vi "Extract Parameters from Comments.vi"(10 "Scan names":string[](array[string]), 11 "Comments":string) -> (1 "Numeric 3":dbl, 2 "Numeric 2":dbl, 3 "Numeric 1":dbl)   [LabVIEW 2020, in "Retrieve and Visualize.lvclass"]
uses:
  Retrieve and Visualize.lvclass
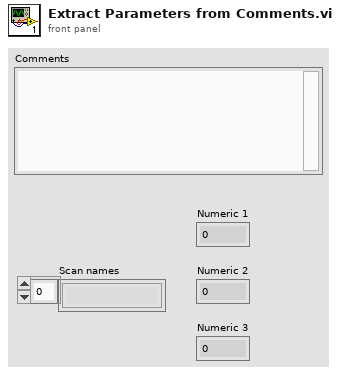
[diagram p1: front panel]
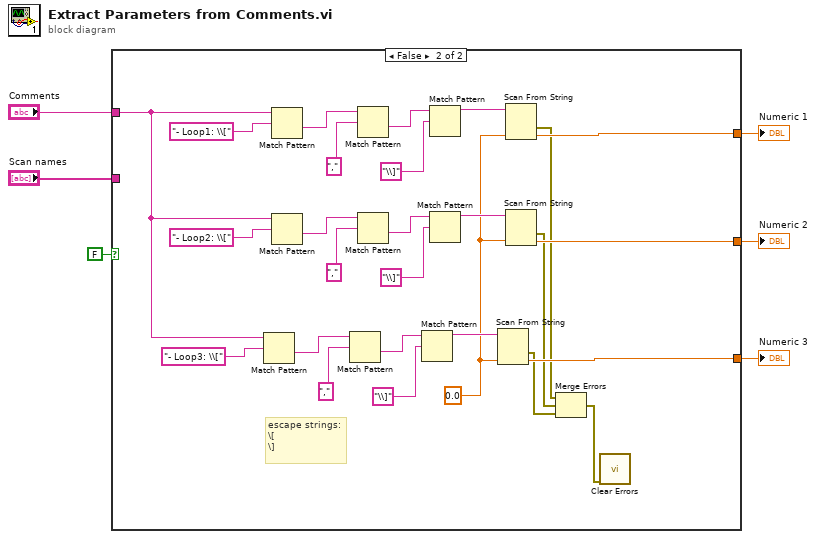
[diagram p0: block diagram]
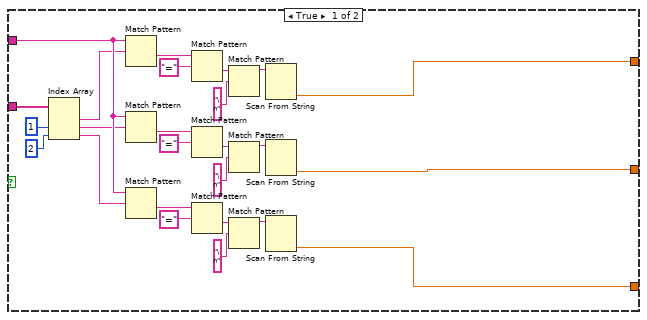
[diagram p2: hidden frame]
diagram:
  n1 = case shown="False" FALSE {
    tunnel: "Scan names" -> [w31 _]
    tunnel: "Comments" -> [w30 w40]
    tunnel: [w29 w39] -> w4
    tunnel: [w28 w38] -> w3
    tunnel: [w27 w37] -> w2
    frame True {
      n2 = Index Array(array=w31, index #2=1 ("index"), index #3=2 ("index")) -> (element #1=w23:string, element #2=w25:string, element #3=w26:string)  [unwired: 1 in]
      n3 = Match Pattern(string=w30, regular expression=w23) -> (after substring=w13:string)  [unwired: 1 in, 3 out]
      n4 = Match Pattern(string=w30, regular expression=w25) -> (after substring=w20:string)  [unwired: 1 in, 3 out]
      n5 = Match Pattern(string=w30, regular expression=w26) -> (after substring=w15:string)  [unwired: 1 in, 3 out]
      n6 = Match Pattern(string=w13, regular expression="=") -> (after substring=w24:string)  [unwired: 1 in, 3 out]
      n7 = Match Pattern(string=w20, regular expression="=") -> (after substring=w22:string)  [unwired: 1 in, 3 out]
      n8 = Match Pattern(string=w15, regular expression="=") -> (after substring=w17:string)  [unwired: 1 in, 3 out]
      n9 = Match Pattern(string=w24, regular expression="\n") -> (before substring=w12:string)  [unwired: 1 in, 3 out]
      n10 = Match Pattern(string=w22, regular expression="\n") -> (before substring=w19:string)  [unwired: 1 in, 3 out]
      n11 = Match Pattern(string=w17, regular expression="\n") -> (before substring=w11:string)  [unwired: 1 in, 3 out]
      n12 = Scan From String(input string=w12) -> (output 1=w28:dbl)  [unwired: 4 in, 3 out]
      n13 = Scan From String(input string=w19) -> (output 1=w27:dbl)  [unwired: 4 in, 3 out]
      n14 = Scan From String(input string=w11) -> (output 1=w29:dbl)  [unwired: 4 in, 3 out]
    }
    frame False {
      w33 = 0.0
      # "escape strings:\n\\[\n\\]"
      n15 = Match Pattern(string=w40, regular expression="- Loop3: \\[") -> (after substring=w45:string)  [unwired: 1 in, 3 out]
      n16 = Match Pattern(string=w40, regular expression="- Loop1: \\[") -> (after substring=w57:string)  [unwired: 1 in, 3 out]
      n17 = Match Pattern(string=w40, regular expression="- Loop2: \\[") -> (after substring=w48:string)  [unwired: 1 in, 3 out]
      n18 = Match Pattern(string=w45, regular expression=",") -> (after substring=w44:string)  [unwired: 1 in, 3 out]
      n19 = Match Pattern(string=w57, regular expression=",") -> (after substring=w56:string)  [unwired: 1 in, 3 out]
      n20 = Match Pattern(string=w48, regular expression=",") -> (after substring=w49:string)  [unwired: 1 in, 3 out]
      n21 = Match Pattern(string=w44, regular expression="\\]") -> (before substring=w43:string)  [unwired: 1 in, 3 out]
      n22 = Match Pattern(string=w56, regular expression="\\]") -> (before substring=w55:string)  [unwired: 1 in, 3 out]
      n23 = Match Pattern(string=w49, regular expression="\\]") -> (before substring=w50:string)  [unwired: 1 in, 3 out]
      n24 = Scan From String(input string=w43, default 1=w33) -> (error out=w34:errorcluster, output 1=w39:dbl)  [unwired: 3 in, 2 out]
      n25 = Scan From String(input string=w55, default 1=w33) -> (error out=w36:errorcluster, output 1=w38:dbl)  [unwired: 3 in, 2 out]
      n26 = Scan From String(input string=w50, default 1=w33) -> (error out=w35:errorcluster, output 1=w37:dbl)  [unwired: 3 in, 2 out]
      n27 = Merge Errors(w36, w35, w34) -> (w32:errorcluster)
      n28 = call <vilib>:"Clear Errors.vi"("error in (no error)"=w32) -> ()  [unwired: 5 in, 2 out]
    }
  }
  "Numeric 3" <- w4
  "Numeric 1" <- w3
  "Numeric 2" <- w2
